vi "Write2DDblArray.vi"(10 "Write":dbl[][](array[numeric]), 11 "Name":string) -> (0 "error out":errorcluster, 3 "Overwrote":bool=TRUE)   [LabVIEW 2014]
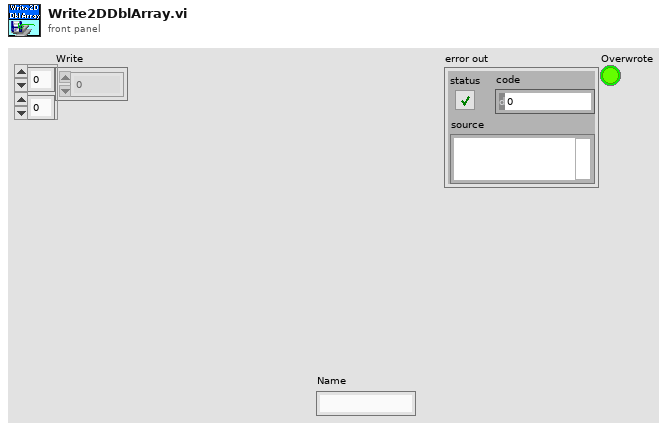
[diagram p1: front panel]
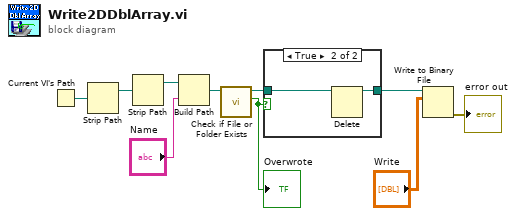
[diagram p0: block diagram]
diagram:
  n1 = Current VI's Path() -> (path=w10:path)
  n2 = Strip Path(path=w10) -> (stripped path=w9:path)  [unwired: 1 out]
  n3 = Strip Path(path=w9) -> (stripped path=w8:path)  [unwired: 1 out]
  n4 = Build Path(base path=w8, name or relative path="Name") -> (appended path=w6:path)
  n5 = call <vilib>:"Check if File or Folder Exists.vi"("path"=w6) -> ("file or folder exists?"=w2:bool, "dup path"=w5:path)  [unwired: 8 in, 1 out]
  "Overwrote" <- w2
  n6 = case shown="True" w2 {
    tunnel: w5 -> [w11 w13]
    tunnel: [w11 w12] -> w3
    frame False {
    }
    frame True {
      n7 = Delete(path (use dialog)=w13) -> (deleted path=w12:path)  [unwired: 4 in, 2 out]
    }
  }
  n8 = Write to Binary File(file (use dialog)=w3, data="Write") -> (error out=→"error out":errorcluster)  [unwired: 4 in, 2 out]
